vi "XY Graph Add Single Plot with Name.vi"(0 "XYGraph Ref in":T4, 1 "Scales (Default)":T3, 2 "Plot Interpolation (Previous Plot's Style)":T2=enum."Use Previous Plot's Style", 3 "Keep Existing Plots (T)":bool=TRUE, 5 "Plot":cluster{"X Array":dbl[], "Y Array":dbl[]}, 7 "Plot Metadata":variant, 9 "Plot Name (\"Plot\")":string, 11 "error in (no error)":errorcluster, 13 "Plot Color (Default)":u32(colorbox)=15781887, 14 "Point Style (Dot)":T1=enum."Dot") -> (4 "XY Graph Caption (or Label)":string, 8 "Plot Index":i32, 10 "Plot Name":string, 15 "error out":errorcluster)   [LabVIEW 2021, in "XY Graph Add-Ons.lvlib"]
uses:
  XY Graph Add-Ons.lvlib
  XY Graph Refnum.ctl
  Plot Scales.ctl
  LabVIEW Plot Interpolation.ctl
  Plot Point Style.ctl
  Plot Magic Color (Unchanged).ctl
  XY Graph Get Plots Metadata.vi
  XY Graph Set Plots Metadata.vi
  XY Graph Get Max Legend Size.vi
  Strings/Strings.lvlib
  Graphs.lvlib
  Error/Error.lvlib
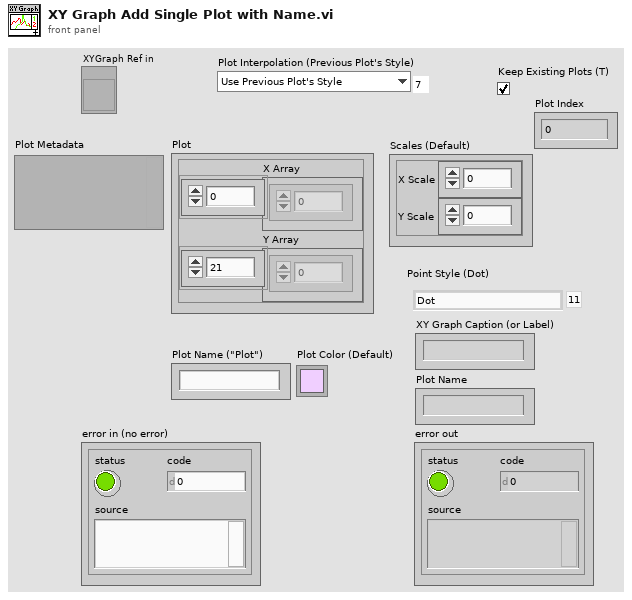
[diagram p1: front panel]
types:
  T1 = typedef "Graphs.lvlib/Plot Point Style.ctl" = enum16{"not defined", "None", "Empty Circle", "Filled Circle", "Thick Circle", "Dotted Circle", "Empty Square", "Filled Square", "Thick Square", "Dotted Square", "Small Filled Square", "Dot", "Cross", "Tiny Cross", "Large X", "Small x", "Diamond", "Small Empty Square"}
  T2 = typedef "Graphs.lvlib/LabVIEW Plot Interpolation.ctl" = enum16{"Point (.)", "Stepwise Right (--.)", "Line + Point (\\. /)", "Stepwise Left (.--)", "Stepwise Centered (-.-)", "Stepwise Vertical (|.|)", "Line (-)", "Use Previous Plot's Style"}
  T3 = typedef "XY Graph Add-Ons.lvlib/Plot Scales.ctl" = cluster{"X Scale":u32, "Y Scale":u32}
  T4 = typedef "XY Graph Add-Ons.lvlib/XY Graph Refnum.ctl" = refnum<vi>
  T5 = typedef "Graphs.lvlib/Plot Magic Color (Unchanged).ctl" = u32
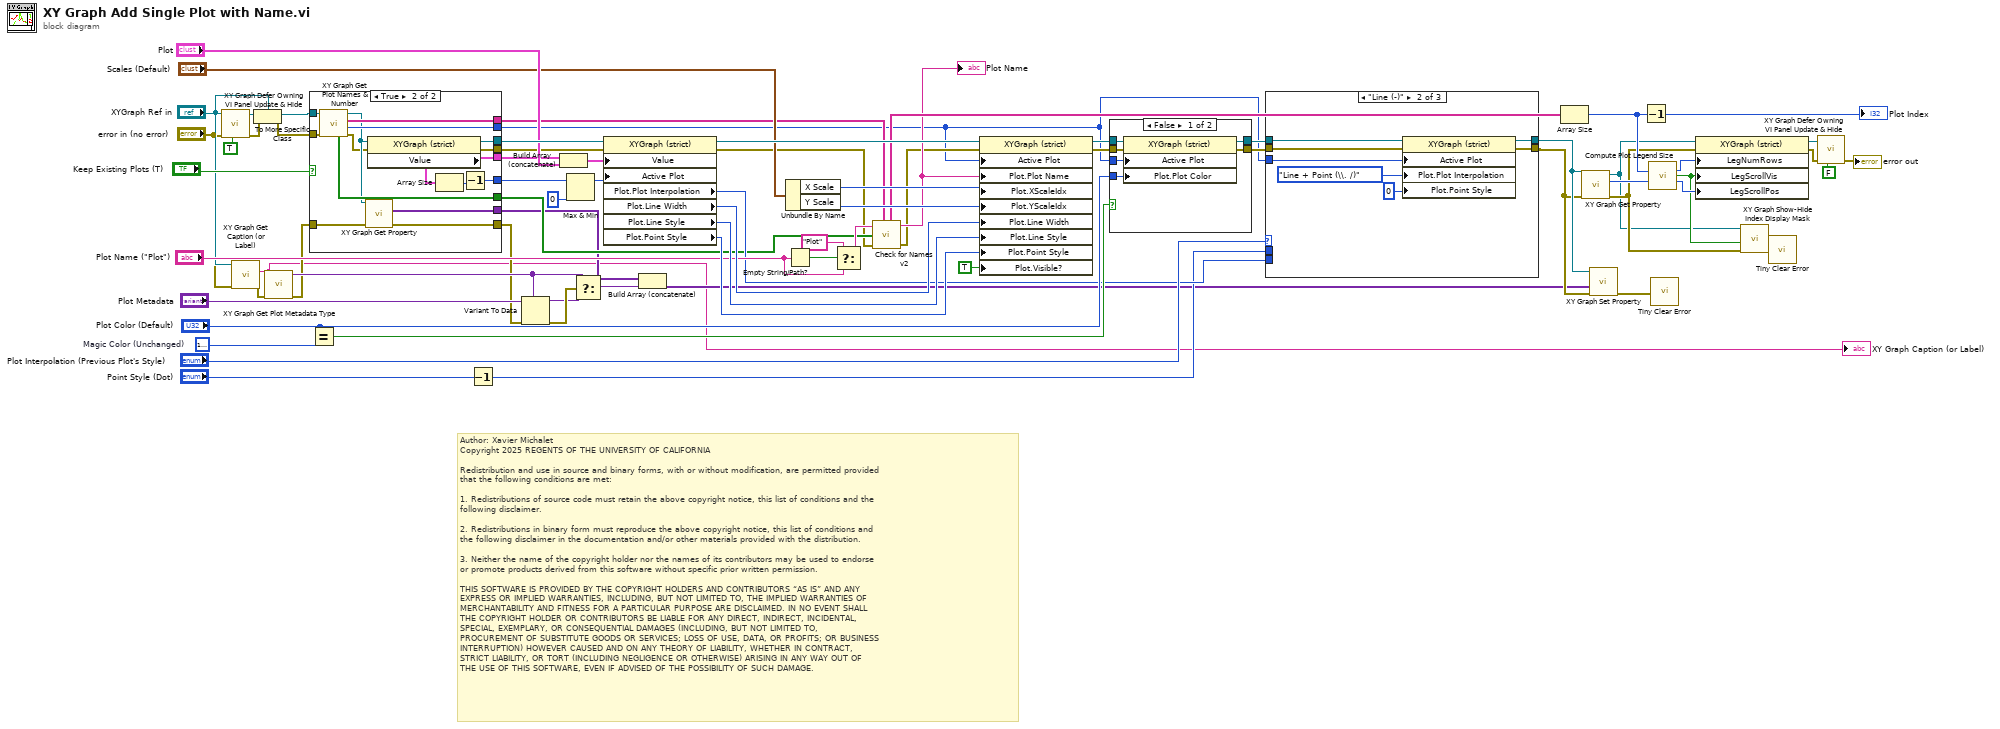
[diagram p0: block diagram]
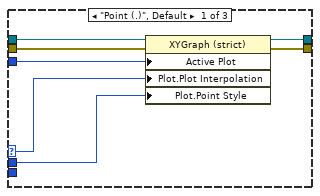
[diagram p3: hidden frame]
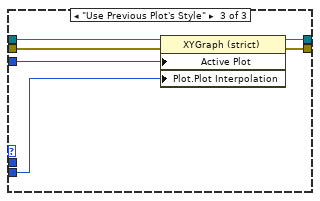
[diagram p4: hidden frame]
diagram:
  w58 = T5 15781887  # Magic Color (Unchanged)
  # "Author: Xavier Michalet\nCopyright 2025 REGENTS OF THE UNIVERSITY OF CALIFORNIA\n\nRedistribution and use in source and binary forms, with or without modification, are permitted provided\nthat the following conditions are met:\n\n1. Redistributions of source code must retain the above copyright notice, this list of conditions and the\nfollowing disclaimer.\n\n2. Redistributions in binary form must reproduce the above copyright notice, this list of conditions and\nthe following disclaimer in the documentation and/or other materials provided with the distribution.\n\n3. Neither the name of the copyright holder nor the names of its contributors may be used to endorse \nor promote products derived from this software without specific prior written permission.\n\nTHIS SOFTWARE IS PROVIDED BY THE COPYRIGHT HOLDERS AND CONTRIBUTORS “AS IS” AND ANY \nEXPRESS OR IMPLIED WARRANTIES, INCLUDING, BUT NOT LIMITED TO, THE IMPLIED WARRANTIES OF\nMERCHANTABILITY AND FITNESS FOR A PARTICULAR PURPOSE ARE DISCLAIMED. IN NO EVENT SHALL\nTHE COPYRIGHT HOLDER OR CONTRIBUTORS BE LIABLE FOR ANY DIRECT, INDIRECT, INCIDENTAL, \nSPECIAL, EXEMPLARY, OR CONSEQUENTIAL DAMAGES (INCLUDING, BUT NOT LIMITED TO, \nPROCUREMENT OF SUBSTITUTE GOODS OR SERVICES; LOSS OF USE, DATA, OR PROFITS; OR BUSINESS\nINTERRUPTION) HOWEVER CAUSED AND ON ANY THEORY OF LIABILITY, WHETHER IN CONTRACT, \nSTRICT LIABILITY, OR TORT (INCLUDING NEGLIGENCE OR OTHERWISE) ARISING IN ANY WAY OUT OF\nTHE USE OF THIS SOFTWARE, EVEN IF ADVISED OF THE POSSIBILITY OF SUCH DAMAGE."
  n1 = call "XY Graph Defer Owning VI Panel Update & Hide.vi"("Defer Owning Panel Update"=TRUE, "error in (no error)"="error in (no error)", "XY Graph Refnum in"="XYGraph Ref in") -> ("error out"=w30:errorcluster, "XY Graph Refnum out"=w37:refnum<vi>)  [unwired: 7 in]
  n2 = call "XY Graph Get Caption (or Label).vi"("error in (no error)"="error in (no error)", "XY Graph in"="XYGraph Ref in") -> ("error out"=w7:errorcluster, "Caption (or Label) Text"=w6:string)  [unwired: 7 in, 1 out]
  "XY Graph Caption (or Label)" <- w6
  n3 = To More Specific Class(target class="XYGraph Ref in", reference=w37, error in=w30) -> (specific class reference=w31:T4, error out=w29:errorcluster)
  n4 = call "XY Graph Get Plot Metadata Type.vi"("Error In"=w7, "Graph Label"=w6) -> ("Error Out"=w10:errorcluster, "Plot Metadata Type"=w13:variant)  [unwired: 7 in, 1 out]
  n5 = case shown="True" "Keep Existing Plots (T)" {
    tunnel: w31 -> [w76 w91]
    tunnel: [w76 w90] -> w72
    tunnel: w29 -> [w75 w89]
    tunnel: [_ w88] -> w69
    tunnel: [_ w86] -> w68
    tunnel: [_ w85] -> w43
    tunnel: [_ w84] -> w1
    tunnel: [w75 w83] -> w47
    tunnel: [_ w82] -> w34
    tunnel: [_ w79] -> w19
    tunnel: w10 -> [w74 w78]
    tunnel: [w74 w77] -> w9
    frame False {
    }
    frame True {
      n6 = call "XY Graph Get Plot Names & Number.vi"("error in (no error)"=w89, "XYGraph in"=w91) -> ("error out"=w80:errorcluster, "# Plots"=w84:i32, "Plot Names"=w85:string[], "XYGraph out"=w81:T4, "Empty Plots?"=w82:bool[])  [unwired: 4 in, 1 out]
      n7 = call-poly "XY Graph Get Property.vi"("Error In"=w78, "XYGraph Ref"=w81) -> ("Error Out"=w77:errorcluster, "Plot Metadata"=w79:variant[])  [unwired: 6 in, 2 out]
      n8 = property class="XYGraph (strict)"(reference=w81, error in=w80) -> (reference out=w90:T4, error out=w83:errorcluster, "Value"=w88:cluster{"X Array":dbl[], "Y Array":dbl[]}[])
      n9 = Array Size(array=w88) -> (size(s)=w87:i32)
      n10 = Decrement(x=w87) -> (x-1=w86:i32)
    }
  }
  n11 = Equal?(x="Plot Color (Default)", y=w58) -> (x = y?=w55:bool)
  n12 = Decrement(x="Point Style (Dot)") -> (x-1=w39:T1)
  n13 = Variant To Data(error in=w9, type=w13, Variant="Plot Metadata") -> (data=w12:variant, error out=w14:errorcluster)
  n14 = Build Array (concatenate)(w69, "Plot") -> (w73:cluster{"X Array":dbl[], "Y Array":dbl[]}[])
  n15 = Max & Min(x=w68, y=0) -> (max(x,y)=w49:i32)  [unwired: 1 out]
  n16 = Select(t=w13, s=w14, f=w12) -> (s? t:f=w11:variant)
  n17 = property class="XYGraph (strict)"(reference=w72, error in=w47, "Value"=w73, "Active Plot"=w49) -> (reference out=w71:T4, error out=w33:errorcluster, "Plot.Plot Interpolation"=w50:u8, "Plot.Line Width"=w67:u8, "Plot.Line Style"=w66:u8, "Plot.Point Style"=w65:u8)
  n18 = Build Array (concatenate)(w19, w11) -> (w18:variant[])
  n19 = Unbundle By Name("Scales (Default)") -> ("X Scale"=w64:u32, "Y Scale"=w63:u32)
  n20 = Empty String/Path?(string/path="Plot Name (\"Plot\")") -> (empty?=w62:bool)
  n21 = Select(t="Plot", s=w62, f="Plot Name (\"Plot\")") -> (s? t:f=w41:string)
  n22 = call "Check for Names v2.vi"("New Name"=w41, "Name List"=w43, "Empty Plots?"=w34, "Error In"=w33) -> ("New Name List"=w42:string[], "New Name"=w40:string, "Error Out"=w32:errorcluster)  [unwired: 2 in, 1 out]
  "Plot Name" <- w40
  n23 = property class="XYGraph (strict)"(reference=w71, error in=w32, "Active Plot"=w1, "Plot.Plot Name"=w40, "Plot.XScaleIdx"=w64, "Plot.YScaleIdx"=w63, "Plot.Line Width"=w67, "Plot.Line Style"=w66, "Plot.Point Style"=w65, "Plot.Visible?"=TRUE ("Plot.Visible")) -> (reference out=w57:T4, error out=w56:errorcluster)
  n24 = case shown="False" w55 {
    tunnel: w57 -> [w97 w99]
    tunnel: [w96 w99] -> w53
    tunnel: w56 -> [w95 w98]
    tunnel: [w94 w98] -> w52
    tunnel: w1 -> [w93 _]
    tunnel: "Plot Color (Default)" -> [w92 _]
    frame False {
      n25 = property class="XYGraph (strict)"(reference=w97, error in=w95, "Active Plot"=w93, "Plot.Plot Color"=w92) -> (reference out=w96:T4, error out=w94:errorcluster)
    }
    frame True {
    }
  }
  n26 = case shown="\"Line (-)\"" "Plot Interpolation (Previous Plot's Style)" {
    selector: "Plot Interpolation (Previous Plot's Style)" -> [w101 _ _]
    tunnel: w53 -> [w106 w113 w119]
    tunnel: [w105 w112 w118] -> w21
    tunnel: w52 -> [w104 w111 w117]
    tunnel: [w103 w110 w116] -> w20
    tunnel: w1 -> [w102 w109 w115]
    tunnel: w50 -> [_ _ w114]
    tunnel: w39 -> [w100 _ _]
    frame "Point (.)", Default {
      n27 = property class="XYGraph (strict)"(reference=w106, error in=w104, "Active Plot"=w102, "Plot.Plot Interpolation"=w101, "Plot.Point Style"=w100) -> (reference out=w105:T4, error out=w103:errorcluster)
    }
    frame "Line (-)" {
      n28 = property class="XYGraph (strict)"(reference=w113, error in=w111, "Active Plot"=w109, "Plot.Plot Interpolation"=LabVIEW_Plot_Interpolation."Line + Point (\\. /)" ("Plot Interpolation (Previous Plot's Style)"), "Plot.Point Style"=u8 0) -> (reference out=w112:T4, error out=w110:errorcluster)
    }
    frame "Use Previous Plot's Style" {
      n29 = property class="XYGraph (strict)"(reference=w119, error in=w117, "Active Plot"=w115, "Plot.Plot Interpolation"=w114) -> (reference out=w118:T4, error out=w116:errorcluster)
    }
  }
  n30 = Array Size(array=w42) -> (size(s)=w27:i32)
  n31 = call-poly "XY Graph Get Property.vi"("Error In"=w20, "XYGraph Refnum"=w21) -> ("Error Out"=w3:errorcluster, "Max Legend Size"=w28:i32, "XYGraph Refnum"=w2:T4)  [unwired: 6 in, 1 out]
  n32 = call-poly "XY Graph Set Property.vi"("error in (no error)"=w20, "Plots Metadata"=w18, "XY Graph Refnum"=w21) -> ("error out"=w17:errorcluster)  [unwired: 7 in, 1 out]
  n33 = Decrement(x=w27) -> (x-1=→"Plot Index":i32)
  n34 = call "Compute Plot Legend Size.vi"("# Plots"=w27, "Max Legend Size"=w28) -> ("LegNumRows"=w26:u32, "LegScrollVis"=w4:bool, "LegScrollPos"=w25:u32)  [unwired: 11 in]
  n35 = call "Tiny Clear Error.vi"("Error In"=w17) -> ()  [unwired: 8 in, 1 out]
  n36 = property class="XYGraph (strict)"(reference=w2, error in=w3, "LegNumRows"=w26, "LegScrollVis"=w4, "LegScrollPos"=w25) -> (reference out=w22:T4, error out=w35:errorcluster)
  n37 = call "XY Graph Show-Hide Index Display Mask.vi"("error in (no error)"=w3, "Show(T)/Hide(F)"=w4, "XYGraph Ref"=w2) -> ("error out"=w5:errorcluster)  [unwired: 7 in, 1 out]
  n38 = call "Tiny Clear Error.vi"("Error In"=w5) -> ()  [unwired: 8 in, 1 out]
  n39 = call "XY Graph Defer Owning VI Panel Update & Hide.vi"("Defer Owning Panel Update"=FALSE, "error in (no error)"=w35, "XY Graph Refnum in"=w22) -> ("error out"=→"error out":errorcluster)  [unwired: 7 in, 1 out]
